vi "Get BC.vi"(8 "error in (no error)":errorcluster, 10 "Domain":refnum<class "NI_Domain.lvclass">, 11 "BC_Evolut_1D_VIRef in":refnum<class "NI_BC_Evolut_1D_VIRef.lvclass">) -> (0 "error out":errorcluster, 2 "BC":variant, 3 "BC_Evolut_1D_VIRef out":refnum<class "NI_BC_Evolut_1D_VIRef.lvclass">)   [LabVIEW 2017, in "NI_PDE.lvlib" / "NI_BC_Evolut_1D_VIRef.lvclass"]
uses:
  <vilib>/gmath/pde.llb/BCClass/BC_Evolut_1D_VIRef/NI_BC_Evolut_1D_VIRef.lvclass
  <vilib>/gmath/pde.llb/DomainClass/NI_Domain.lvclass
  <vilib>/gmath/pde.llb/BCClass/BC_Evolut_1D_VIRef/BC Data.ctl
  <vilib>/gmath/pde.llb/Common/PDE_BC Type.ctl
  <vilib>/gmath/pde.llb/Common/PDE_BC Position 1D.ctl
  <vilib>/gmath/pde.llb/BCClass/BC_Evolut_1D_VIRef/NI_BC_Evolut_1D_VIRef.lvclass/NI_BC_Evolut_1D_VIRef.ctl
  <vilib>/gmath/NI_PDE.lvlib
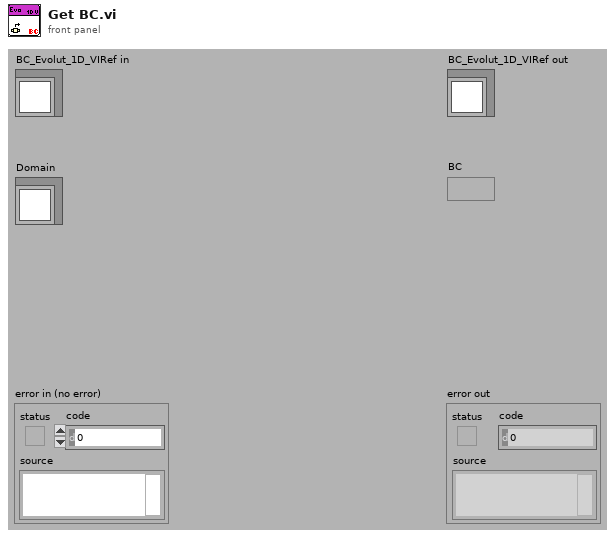
[diagram p1: front panel]
types:
  T1 = typedef "NI_PDE.lvlib/NI_BC_Evolut_1D_VIRef.lvclass/BC Data.ctl" = cluster{"type":T2, "position":T3, "G":refnum<vi>, "data":variant}
  T2 = typedef "NI_PDE.lvlib/PDE_BC Type.ctl" = i32
  T3 = typedef "NI_PDE.lvlib/PDE_BC Position 1D.ctl" = i32
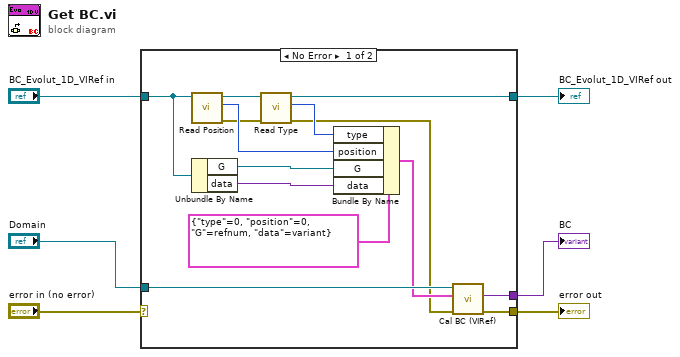
[diagram p0: block diagram]
diagram:
  n1 = case shown="No Error" "error in (no error)" {
    selector: "error in (no error)" -> [_ w21]
    tunnel: "BC_Evolut_1D_VIRef in" -> [w15 w22]
    tunnel: [w19 _] -> w3
    tunnel: [w16 w22] -> w6
    tunnel: [w18 w21] -> w4
    tunnel: "Domain" -> [w20 _]
    frame No Error {
      n2 = call-dynamic "Read Position.vi"("BC_Evolut_1D.lvclass in"=w15) -> ("error out"=w8:errorcluster, "BC position 1D"=w12:T3, "BC_Evolut_1D.lvclass out"=w17:refnum<class "NI_BC_Evolut_1D_VIRef.lvclass">)  [unwired: 1 in, 7 out]
      n3 = Unbundle By Name(w15) -> ("G"=w11:refnum<vi>, "data"=w10:variant)
      n4 = call-dynamic "Read Type.vi"("error in (no error)"=w8, "BC.lvclass in"=w17) -> ("error out"=w7:errorcluster, "BC type"=w13:T2, "BC.lvclass out"=w16:refnum<class "NI_BC_Evolut_1D_VIRef.lvclass">)  [unwired: 7 out]
      n5 = Bundle By Name(cluster=T1 {"type"=0, "position"=0, "G"=refnum, "data"=variant} ("BC data"), "type"=w13, "position"=w12, "G"=w11, "data"=w10) -> (w9:T1)
      n6 = call-dynamic "Cal BC (VIRef).vi"("error in (no error)"=w7, "BC in"=w9, "Domain in"=w20) -> ("error out"=w18:errorcluster, "BC out"=w19:variant)  [unwired: 7 out]
    }
    frame Error {
    }
  }
  "BC" <- w3
  "error out" <- w4
  "BC_Evolut_1D_VIRef out" <- w6
